vi "Vxmdriverlv8.Vi"(0 "Port":i32=1 min=1 max=255 step=1, 1 "Baud Rate":i32=9600 min=9600 max=38400 step=9600, 2 "Open Port":bool, 3 "Close Port":bool, 4 "Clear chars\nfrom port":bool, 5 "Count chars\nat port":bool, 7 "Send\nchars\nto port":bool, 8 "Is Port Open":bool, 9 "Chars to send":string, 11 "Read\nfrom\nport":bool, 12 "Search\nfor\nchars":bool, 14 "Chars to find":string, 15 "Remove\nfrom\nport":bool, 17 "Chars to remove":string, 18 "Hide Terminal":bool, 19 "Show Terminal":bool, 20 "Get\nMotor\nPosition":bool, 21 "Motor\nNumber":i32=1 min=1 max=4 step=1, 24 "Wait\nfor \nchar":bool, 25 "Char(s) to wait for":string, 26 "Char\nTimeout\nTime (ms)":i32=1 min=1 step=1) -> (6 "# chars at port":dbl, 10 "Port\nOpen\nStatus":bool, 13 "Port chars":string, 16 "Chars\nfound":bool, 22 "Motor Position":string, 27 "Char\nto wait\nfor found":bool)   [LabVIEW 2013]
uses:
  Vxmdriver.Dll
panel:
  out "Motor\nPosition\nfunctioned\ncorrectly":bool
  out "Chars\nremoved\ncorrectly":bool
  out "Terminal \nshown\ncorrectly":bool
  out "Terminal \nhid correctly":bool
  out "Chars\nsent \ncorrectly":bool
  out "Chars cleared\ncorrectly":bool
  out "Port\nStatus":bool
  # "Port Functions"
  # "True"
  # "True"
  # "False"
  # "False"
  # "Clear Port"
  # "True"
  # "False"
  # "True"
  # "False"
  # "True"
  # "False"
  # "True"
  # "False"
  # "True"
  # "False"
  # "True"
  # "False"
  # "True"
  # "False"
  # "True"
  # "False"
  # "True"
  # "False"
  # "True"
  # "False"
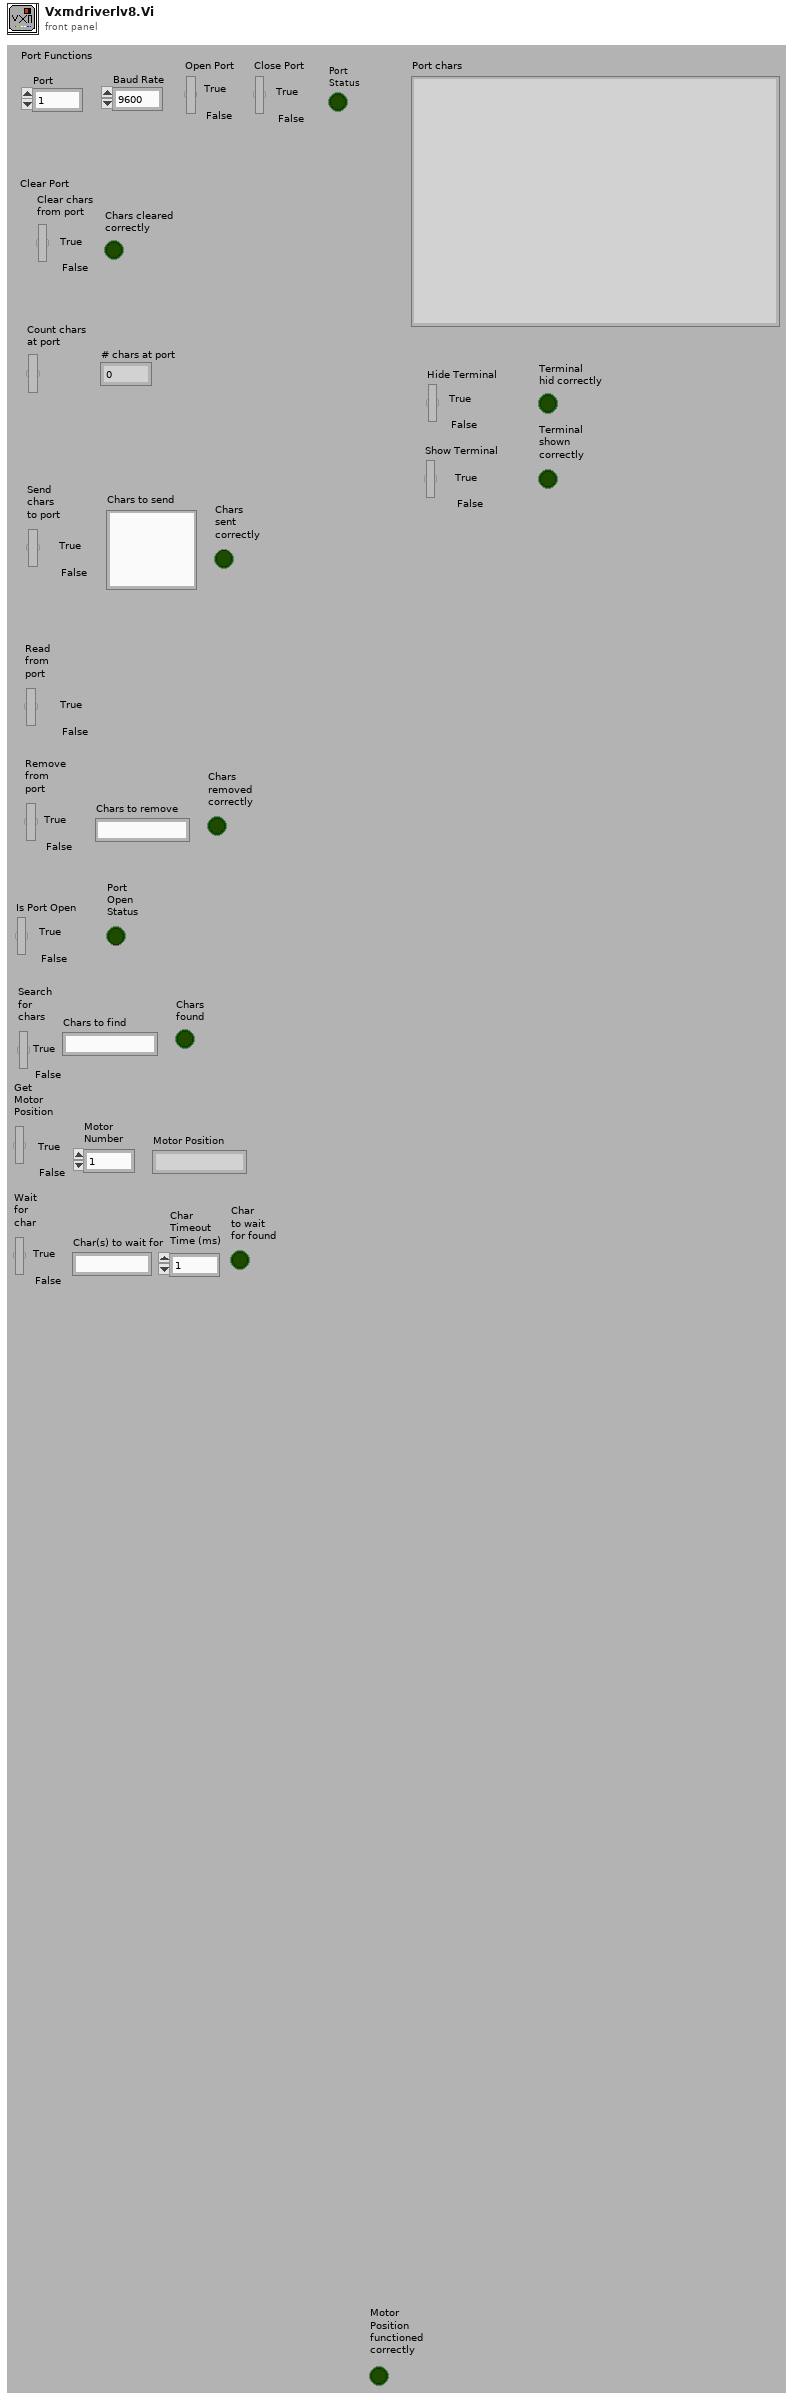
[diagram p1: front panel]
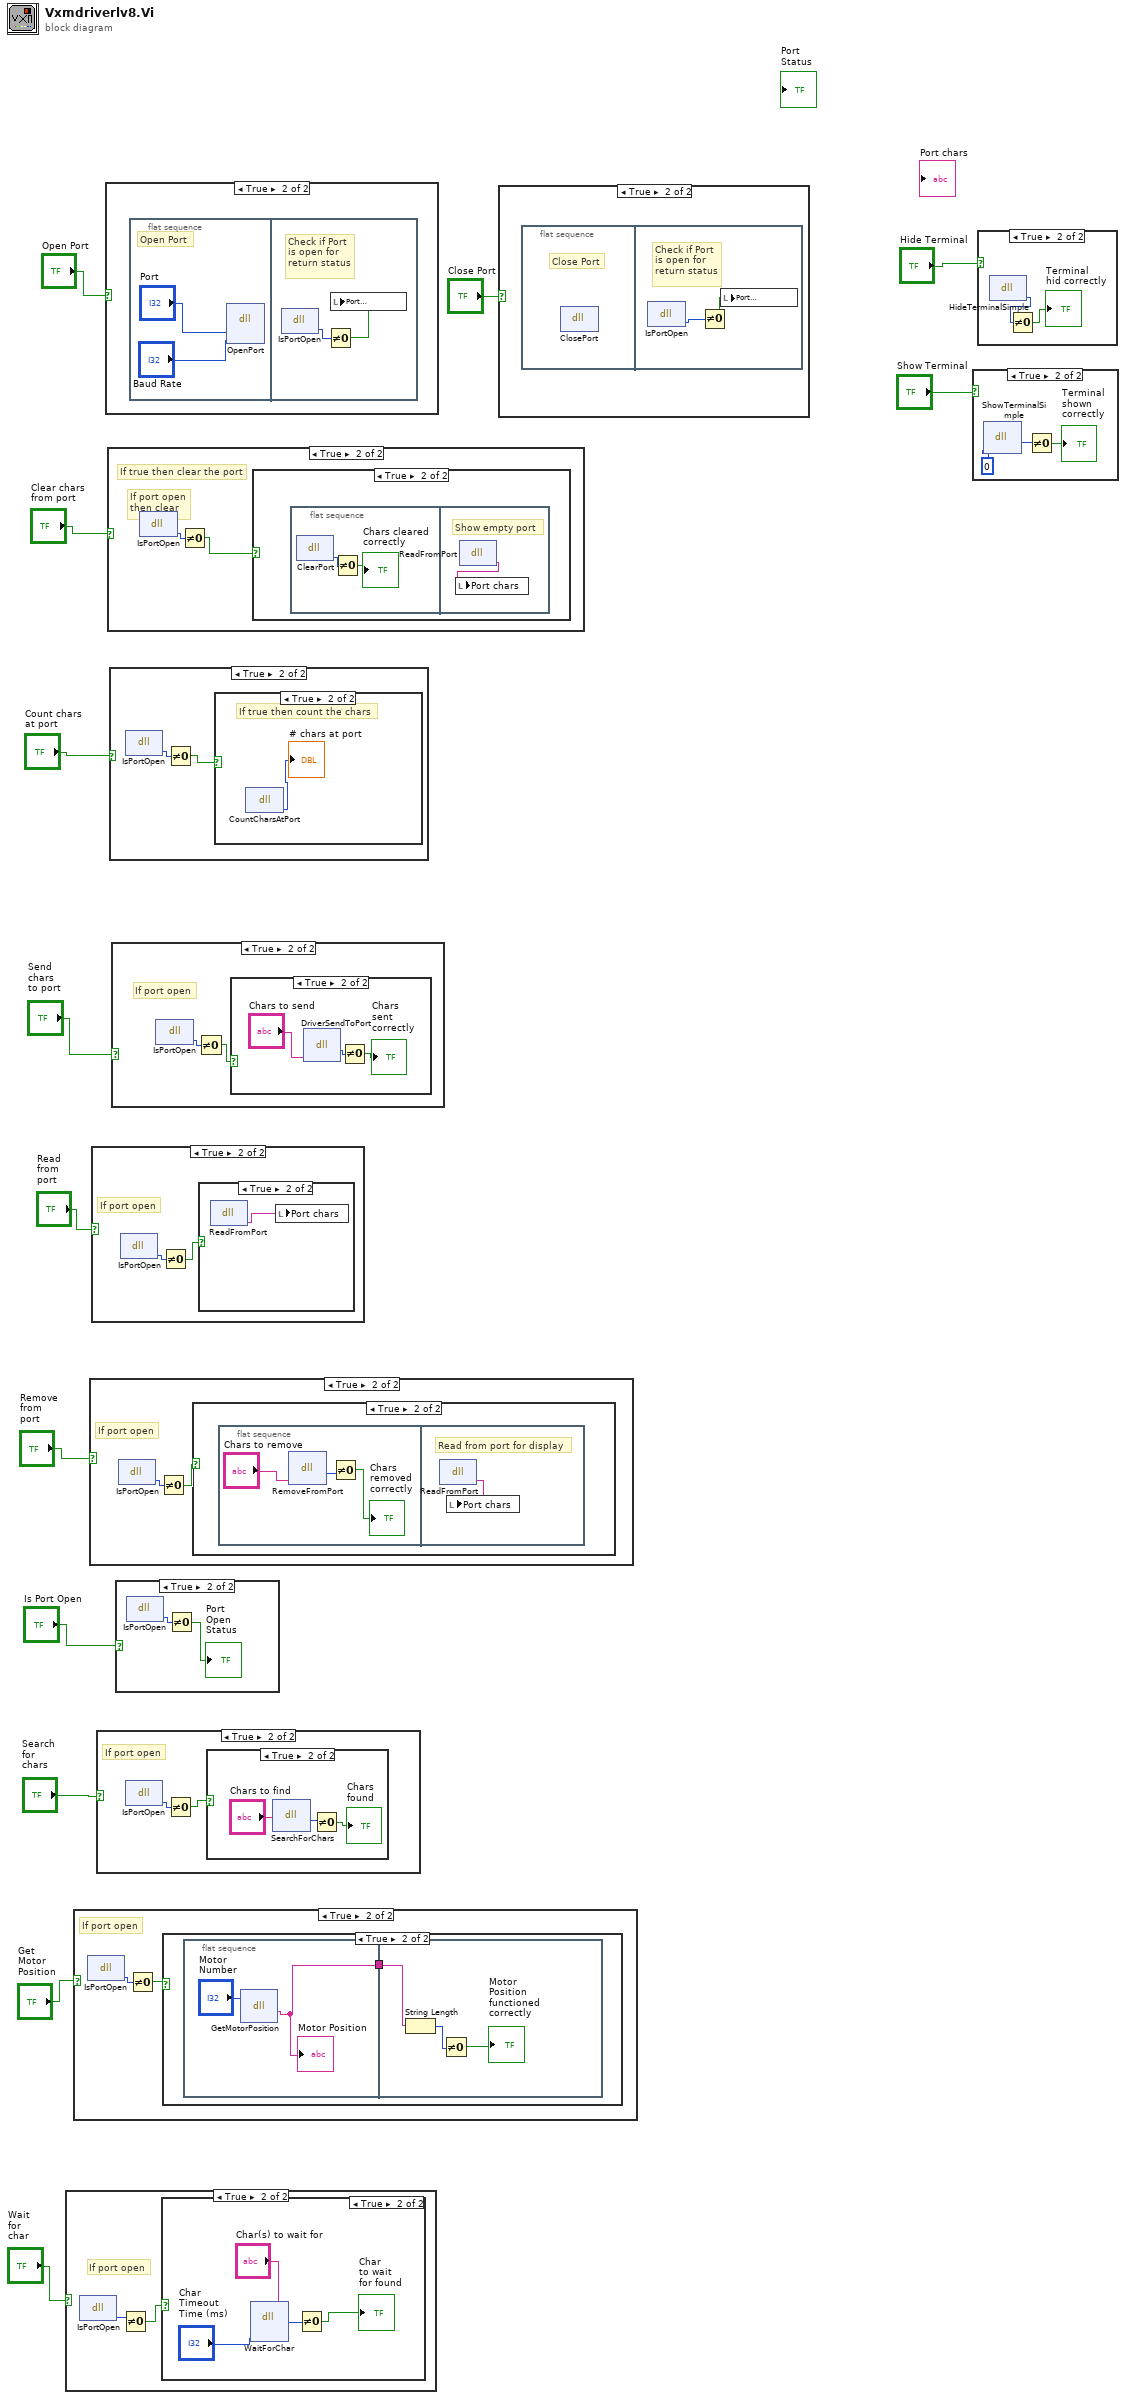
[diagram p0: block diagram]
diagram:
  n1 = case shown="True" "Wait\nfor \nchar" {
    frame False {
    }
    frame True {
      # "If port open"
      n2 = dll-call lib="C:/Users/loasis/COSMOS/Examples/NationalInstruments/vxm_example_lv8/Source/Driver/VxmDriver.dll" fn="IsPortOpen"() -> (w15:i32)  [unwired: 3 in, 2 out]
      n3 = Not Equal To 0?(x=w15) -> (x != 0?=w14:bool)
      n4 = case shown="True" w14 {
        frame False {
        }
        frame True {
          n5 = dll-call lib="C:/Users/loasis/COSMOS/Examples/NationalInstruments/vxm_example_lv8/Source/Driver/VxmDriver.dll" fn="WaitForChar"("CharToWaitFor"="Char(s) to wait for", "TimeOutTime"="Char\nTimeout\nTime (ms)") -> (w17:i32)  [unwired: 5 in, 2 out]
          n6 = Not Equal To 0?(x=w17) -> (x != 0?=→"Char\nto wait\nfor found":bool)
        }
      }
    }
  }
  n7 = case shown="True" "Get\nMotor\nPosition" {
    frame False {
    }
    frame True {
      # "If port open"
      n8 = dll-call lib="C:/Users/loasis/COSMOS/Examples/NationalInstruments/vxm_example_lv8/Source/Driver/VxmDriver.dll" fn="IsPortOpen"() -> (w21:i32)  [unwired: 3 in, 2 out]
      n9 = Not Equal To 0?(x=w21) -> (x != 0?=w20:bool)
      n10 = case shown="True" w20 {
        frame False {
        }
        frame True {
          n11 = flat-sequence {
            tunnel: [w23] -> w22
            tunnel: w22 -> [w25]
            frame #0 {
              n12 = dll-call lib="C:/Users/loasis/COSMOS/Examples/NationalInstruments/vxm_example_lv8/Source/Driver/VxmDriver.dll" fn="GetMotorPosition"("MotorNumber"="Motor\nNumber") -> (w23:string)  [unwired: 4 in, 2 out]
              "Motor Position" <- w23
            }
            frame #1 {
              n13 = String Length(string=w25) -> (length=w27:i32)
              n14 = Not Equal To 0?(x=w27) -> (x != 0?=→"Motor\nPosition\nfunctioned\ncorrectly":bool)
            }
          }
        }
      }
    }
  }
  n15 = case shown="True" "Remove\nfrom\nport" {
    frame False {
    }
    frame True {
      # "If port open"
      n16 = dll-call lib="C:/Users/loasis/COSMOS/Examples/NationalInstruments/vxm_example_lv8/Source/Driver/VxmDriver.dll" fn="IsPortOpen"() -> (w29:i32)  [unwired: 3 in, 2 out]
      n17 = Not Equal To 0?(x=w29) -> (x != 0?=w28:bool)
      n18 = case shown="True" w28 {
        frame False {
        }
        frame True {
          n19 = flat-sequence {
            frame #0 {
              n20 = dll-call lib="C:/Users/loasis/COSMOS/Examples/NationalInstruments/vxm_example_lv8/Source/Driver/VxmDriver.dll" fn="RemoveFromPort"("CharsToRemove"="Chars to remove") -> (w31:i32)  [unwired: 4 in, 2 out]
              n21 = Not Equal To 0?(x=w31) -> (x != 0?=→"Chars\nremoved\ncorrectly":bool)
            }
            frame #1 {
              # "Read from port for display"
              n22 = dll-call lib="C:/Users/loasis/COSMOS/Examples/NationalInstruments/vxm_example_lv8/Source/Driver/VxmDriver.dll" fn="ReadFromPort"() -> (w33:string)  [unwired: 3 in, 2 out]
              n23 = local write "Port chars"(w33) -> ()
            }
          }
        }
      }
    }
  }
  n24 = case shown="True" "Read\nfrom\nport" {
    frame False {
    }
    frame True {
      # "If port open"
      n25 = dll-call lib="C:/Users/loasis/COSMOS/Examples/NationalInstruments/vxm_example_lv8/Source/Driver/VxmDriver.dll" fn="IsPortOpen"() -> (w35:i32)  [unwired: 3 in, 2 out]
      n26 = Not Equal To 0?(x=w35) -> (x != 0?=w34:bool)
      n27 = case shown="True" w34 {
        frame False {
        }
        frame True {
          n28 = dll-call lib="C:/Users/loasis/COSMOS/Examples/NationalInstruments/vxm_example_lv8/Source/Driver/VxmDriver.dll" fn="ReadFromPort"() -> (w36:string)  [unwired: 3 in, 2 out]
          n29 = local write "Port chars"(w36) -> ()
        }
      }
    }
  }
  n30 = case shown="True" "Search\nfor\nchars" {
    frame False {
    }
    frame True {
      # "If port open"
      n31 = dll-call lib="C:/Users/loasis/COSMOS/Examples/NationalInstruments/vxm_example_lv8/Source/Driver/VxmDriver.dll" fn="IsPortOpen"() -> (w38:i32)  [unwired: 3 in, 2 out]
      n32 = Not Equal To 0?(x=w38) -> (x != 0?=w37:bool)
      n33 = case shown="True" w37 {
        frame False {
        }
        frame True {
          n34 = dll-call lib="C:/Users/loasis/COSMOS/Examples/NationalInstruments/vxm_example_lv8/Source/Driver/VxmDriver.dll" fn="SearchForChars"("CharsToFind"="Chars to find") -> (w40:i32)  [unwired: 4 in, 2 out]
          n35 = Not Equal To 0?(x=w40) -> (x != 0?=→"Chars\nfound":bool)
        }
      }
    }
  }
  n36 = case shown="True" "Open Port" {
    frame False {
    }
    frame True {
      n37 = flat-sequence {
        frame #0 {
          # "Open Port"
          n38 = dll-call lib="C:/Users/loasis/COSMOS/Examples/NationalInstruments/vxm_example_lv8/Source/Driver/VxmDriver.dll" fn="OpenPort"("PortNum"="Port", "BaudRate"="Baud Rate") -> ()  [unwired: 6 in, 2 out]
        }
        frame #1 {
          # "Check if Port\nis open for \nreturn status"
          n39 = dll-call lib="C:/Users/loasis/COSMOS/Examples/NationalInstruments/vxm_example_lv8/Source/Driver/VxmDriver.dll" fn="IsPortOpen"() -> (w45:i32)  [unwired: 3 in, 2 out]
          n40 = Not Equal To 0?(x=w45) -> (x != 0?=w44:bool)
          n41 = local write "Port\nStatus"(w44) -> ()
        }
      }
    }
  }
  n42 = case shown="True" "Clear chars\nfrom port" {
    frame False {
    }
    frame True {
      # "If true then clear the port"
      # "If port open\nthen clear"
      n43 = dll-call lib="C:/Users/loasis/COSMOS/Examples/NationalInstruments/vxm_example_lv8/Source/Driver/VxmDriver.dll" fn="IsPortOpen"() -> (w46:i32)  [unwired: 3 in, 2 out]
      n44 = Not Equal To 0?(x=w46) -> (x != 0?=w47:bool)
      n45 = case shown="True" w47 {
        frame False {
        }
        frame True {
          n46 = flat-sequence {
            frame #0 {
              n47 = dll-call lib="C:/Users/loasis/COSMOS/Examples/NationalInstruments/vxm_example_lv8/Source/Driver/VxmDriver.dll" fn="ClearPort"() -> (w48:i32)  [unwired: 3 in, 2 out]
              n48 = Not Equal To 0?(x=w48) -> (x != 0?=→"Chars cleared\ncorrectly":bool)
            }
            frame #1 {
              # "Show empty port"
              n49 = dll-call lib="C:/Users/loasis/COSMOS/Examples/NationalInstruments/vxm_example_lv8/Source/Driver/VxmDriver.dll" fn="ReadFromPort"() -> (w50:string)  [unwired: 3 in, 2 out]
              n50 = local write "Port chars"(w50) -> ()
            }
          }
        }
      }
    }
  }
  n51 = case shown="True" "Count chars\nat port" {
    frame False {
    }
    frame True {
      n52 = dll-call lib="C:/Users/loasis/COSMOS/Examples/NationalInstruments/vxm_example_lv8/Source/Driver/VxmDriver.dll" fn="IsPortOpen"() -> (w52:i32)  [unwired: 3 in, 2 out]
      n53 = Not Equal To 0?(x=w52) -> (x != 0?=w51:bool)
      n54 = case shown="True" w51 {
        frame False {
        }
        frame True {
          # "If true then count the chars"
          n55 = dll-call lib="C:/Users/loasis/COSMOS/Examples/NationalInstruments/vxm_example_lv8/Source/Driver/VxmDriver.dll" fn="CountCharsAtPort"() -> (→"# chars at port":i32)  [unwired: 3 in, 2 out]
        }
      }
    }
  }
  n56 = case shown="True" "Send\nchars\nto port" {
    frame False {
    }
    frame True {
      # "If port open"
      n57 = dll-call lib="C:/Users/loasis/COSMOS/Examples/NationalInstruments/vxm_example_lv8/Source/Driver/VxmDriver.dll" fn="IsPortOpen"() -> (w55:i32)  [unwired: 3 in, 2 out]
      n58 = Not Equal To 0?(x=w55) -> (x != 0?=w54:bool)
      n59 = case shown="True" w54 {
        frame False {
        }
        frame True {
          n60 = dll-call lib="C:/Users/loasis/COSMOS/Examples/NationalInstruments/vxm_example_lv8/Source/Driver/VxmDriver.dll" fn="DriverSendToPort"("VxmCommands"="Chars to send") -> (w57:i32)  [unwired: 4 in, 2 out]
          n61 = Not Equal To 0?(x=w57) -> (x != 0?=→"Chars\nsent \ncorrectly":bool)
        }
      }
    }
  }
  n62 = case shown="True" "Is Port Open" {
    frame False {
    }
    frame True {
      n63 = dll-call lib="C:/Users/loasis/COSMOS/Examples/NationalInstruments/vxm_example_lv8/Source/Driver/VxmDriver.dll" fn="IsPortOpen"() -> (w60:i32)  [unwired: 3 in, 2 out]
      n64 = Not Equal To 0?(x=w60) -> (x != 0?=→"Port\nOpen\nStatus":bool)
    }
  }
  n65 = case shown="True" "Close Port" {
    frame False {
    }
    frame True {
      n66 = flat-sequence {
        frame #0 {
          # "Close Port"
          n67 = dll-call lib="C:/Users/loasis/COSMOS/Examples/NationalInstruments/vxm_example_lv8/Source/Driver/VxmDriver.dll" fn="ClosePort"() -> ()  [unwired: 4 in, 2 out]
        }
        frame #1 {
          # "Check if Port\nis open for \nreturn status"
          n68 = dll-call lib="C:/Users/loasis/COSMOS/Examples/NationalInstruments/vxm_example_lv8/Source/Driver/VxmDriver.dll" fn="IsPortOpen"() -> (w62:i32)  [unwired: 3 in, 2 out]
          n69 = Not Equal To 0?(x=w62) -> (x != 0?=w61:bool)
          n70 = local write "Port\nStatus"(w61) -> ()
        }
      }
    }
  }
  n71 = case shown="True" "Show Terminal" {
    frame False {
    }
    frame True {
      n72 = dll-call lib="C:/Users/loasis/COSMOS/Examples/NationalInstruments/vxm_example_lv8/Source/Driver/VxmDriver.dll" fn="ShowTerminalSimple"("ParentHwnd"=0) -> (w64:i32)  [unwired: 4 in, 2 out]
      n73 = Not Equal To 0?(x=w64) -> (x != 0?=→"Terminal \nshown\ncorrectly":bool)
    }
  }
  n74 = case shown="True" "Hide Terminal" {
    frame False {
    }
    frame True {
      n75 = dll-call lib="C:/Users/loasis/COSMOS/Examples/NationalInstruments/vxm_example_lv8/Source/Driver/VxmDriver.dll" fn="HideTerminalSimple"() -> (w67:i32)  [unwired: 3 in, 2 out]
      n76 = Not Equal To 0?(x=w67) -> (x != 0?=→"Terminal \nhid correctly":bool)
    }
  }
